vi "reward_behavior_michelle_visjitter_conswinadaptive_enticefx.vi"() -> ()   [LabVIEW 2019]
doc: "The myRIO Project template acquires acceleration data from the onboard accelerometer and displays the changes of acceleration values in a waveform chart."
uses:
  <vilib>/Analysis/Matrix/Datatypes/RealMatrix.ctl
  <vilib>/myRIO/Common/Instrument Driver Framework/myRIO v1.0/Encoder/typedefs/Encoder Signal Mode.ctl
  <vilib>/myRIO/Instrument Drivers/Onboard IO/Encoder/typedefs/Encoder Reference.ctl
  <vilib>/myRIO/Common/Instrument Driver Framework/Utilities/typedefs/myRIO Generic Hardware Reference.ctl
  <vilib>/myRIO/Common/Instrument Driver Framework/Utilities/typedefs/Hardware Version Enum.ctl
  <vilib>/myRIO/Common/Instrument Driver Framework/Utilities/typedefs/myRIO v1.0 Reference.ctl
  <vilib>/myRIO/Common/Instrument Driver Framework/Utilities/typedefs/Generic FPGA Reference.ctl
  <vilib>/myRIO/Common/Instrument Driver Framework/myRIO v1.0/Encoder/typedefs/Encoder Channels Enum.ctl
  <vilib>/myRIO/Common/Instrument Driver Framework/myRIO v1.0/Encoder/typedefs/Encoder Configuration v1.0.ctl
  <vilib>/userdefined/High Color/nirio_resource_hc.ctl
  <vilib>/myRIO/Instrument Drivers/Onboard IO/DIO/typedefs/DIO Reference.ctl
  <vilib>/myRIO/Common/Instrument Driver Framework/myRIO v1.0/DIO/typedefs/DIO Channels List.ctl
  <vilib>/myRIO/Common/Instrument Driver Framework/myRIO v1.0/DIO/typedefs/DIO Channels Enum.ctl
  <vilib>/myRIO/Common/Instrument Driver Framework/Utilities/vis/Is FPGA Ref Available.vi
  <vilib>/myRIO/Common/Instrument Driver Framework/myRIO v1.0/Encoder/vis/myRIO v1.1 Open Encoder.vi
  <vilib>/myRIO/Instrument Drivers/Onboard IO/Encoder/vis/Read.vi
  <vilib>/myRIO/Common/Instrument Driver Framework/myRIO v1.0/DIO/vis/myRIO v1.1 Open DIO.vi
  <vilib>/myRIO/Instrument Drivers/Onboard IO/DIO/vis/Write.vi
  <vilib>/myRIO/Instrument Drivers/Onboard IO/DIO/vis/Read.vi
  <vilib>/myRIO/Common/Instrument Driver Framework/Utilities/vis/Validate Channels.vi
  <vilib>/myRIO/Common/Instrument Driver Framework/myRIO v1.0/Encoder/vis/myRIO v1.0 Reserve Encoder.vi
  <vilib>/myRIO/Common/Instrument Driver Framework/myRIO v1.0/DIO/vis/myRIO v1.0 Reserve DIO.vi
  <vilib>/myRIO/Common/Instrument Driver Framework/myRIO v1.0/Encoder/vis/myRIO v1.0 Build MUX Configuration Encoder.vi
  <vilib>/myRIO/Common/Instrument Driver Framework/myRIO v1.0/Resource Manager/vis/myRIO v1.0 Reserve Channel List.vi
  <vilib>/myRIO/Common/Instrument Driver Framework/myRIO v1.0/DIO/vis/myRIO v1.0 Build MUX Configuration DIO.vi
  <vilib>/myRIO/Common/Instrument Driver Framework/myRIO v1.0/Resource Manager/vis/myRIO v1.0 Create Configuration List.vi
  <vilib>/myRIO/Common/Instrument Driver Framework/myRIO v1.0/Resource Manager/vis/myRIO v1.0 Reserve Channel.vi
  <vilib>/myRIO/Common/Instrument Driver Framework/myRIO v1.0/Resource Manager/vis/myRIO v1.0 Unreserve Channel.vi
  <vilib>/myRIO/Common/Instrument Driver Framework/myRIO v1.0/Resource Manager/vis/myRIO v1.0 Build Mutex Name.vi
  <vilib>/Utility/VariantDataType/GetNumericInfo.vi
  <vilib>/Utility/error.llb/Error Cluster From Error Code.vi
  <vilib>/myRIO/Common/Instrument Driver Framework/myRIO v1.0/myRIO v1.1 Open.vi
  <vilib>/myRIO/Common/Instrument Driver Framework/Utilities/vis/IO Manager.vi
  <vilib>/myRIO/Common/Instrument Driver Framework/Utilities/vis/Configuration Manager.vi
  <vilib>/myRIO/Common/Instrument Driver Framework/myRIO v1.0/Resource Manager/vis/myRIO v1.0 Configure IO.vi
  <vilib>/myRIO/Common/Instrument Driver Framework/myRIO v1.0/myRIO v1.0 Close.vi
  <vilib>/myRIO/Common/Instrument Driver Framework/myRIO v1.0/Encoder/vis/myRIO v1.0 Configure Encoder.vi
  <vilib>/myRIO/Common/Instrument Driver Framework/myRIO v1.0/Encoder/vis/myRIO v1.0 Read Encoder.vi
  <vilib>/myRIO/Common/Instrument Driver Framework/myRIO v1.0/DIO/vis/myRIO v1.0 Read DIO.vi
  <vilib>/myRIO/Common/Instrument Driver Framework/myRIO v1.0/DIO/vis/myRIO v1.0 Write DIO.vi
  <vilib>/myRIO/Express VI/Onboard IO/Encoder/Encoder Express VI.xnode
  <vilib>/myRIO/Instrument Drivers/Onboard IO/Encoder/vis/myRIO Encoder Open.xnode
  <vilib>/myRIO/Express VI/Onboard IO/DI/DI Express VI.xnode
  <vilib>/myRIO/Instrument Drivers/Onboard IO/DIO/vis/myRIO DIO Open.xnode
  <vilib>/myRIO/Express VI/Onboard IO/DO/DO Express VI.xnode
  <vilib>/myRIO/Instrument Drivers/Onboard IO/Encoder/Encoder.lvlib
  <vilib>/myRIO/Instrument Drivers/Onboard IO/DIO/DIO.lvlib
  <vilib>/Analysis/Matrix/NI_Matrix.lvlib
panel:
  out "Enticements":i32
  in  "Entice":bool
  out "Misses":i32
  out "GoAhead":bool
  out "TimeOutDuration":i32
  out "ActiveTime":dbl
  out "ConsumptionGo":bool=TRUE
  out "Consumption_Period":i32
  out "Watch_Display":bool=TRUE
  in  "Give reward":bool
  out "Timings":dbl[](array[numeric])
  out "ISI":dbl
  out "ISI start time":dbl
  out "Time_out":bool=TRUE
  out "Time since lick":dbl
  out "Time of last lick":dbl
  out "Rewarded trials":dbl[](array[numeric])
  out "Rewards":u16
  out "Active Trial":bool
  out "Array temp2":T1
  out "Stimuli Loaded":bool
  out "Stim_ID":dbl[](array[numeric])
  out "Reward_mat":dbl[](array[numeric])
  out "Reward":bool=TRUE
  out "Frame clock":i32
  out "Licks":u32
  out "Lick":bool
  out "Time":dbl
  out "Stop":bool
  in  "Frames to collect":u32
  out "Overflow?":bool
  out "Counter Value":i32
  out "Velocity":dbl
  out "Velocity Plot":dbl[](graph)
  out "Velocity array":dbl[](array[numeric])
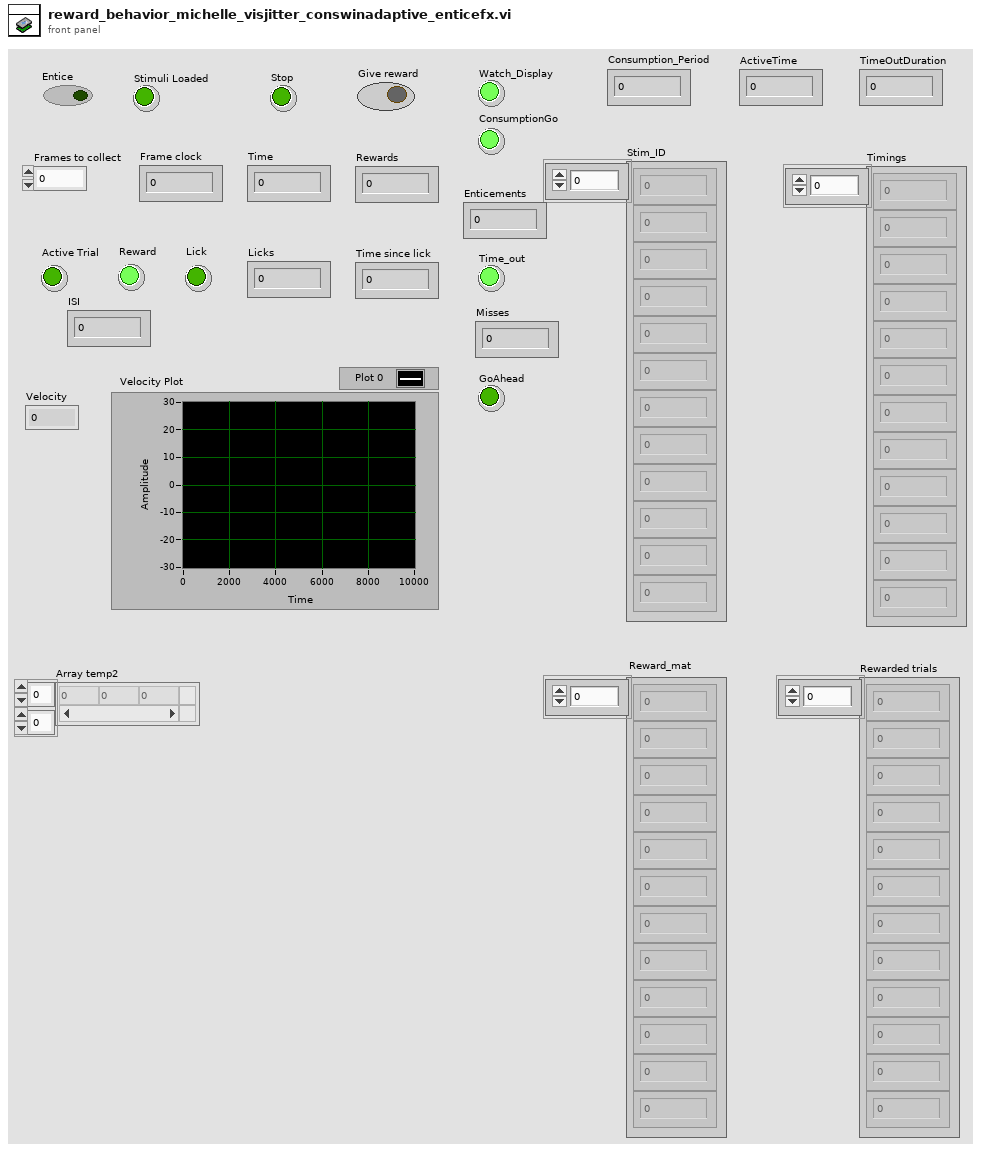
[diagram p1: front panel]
types:
  T1 = typedef "NI_Matrix.lvlib/RealMatrix.ctl" = dbl[][]
  T2 = typedef "Encoder.lvlib/Encoder Reference.ctl" = cluster{"myRIO Reference":T3, "Encoder Channels Enum":T7}
  T3 = typedef "myRIO Generic Hardware Reference.ctl" = cluster{"myRIO Model":T4, "myRIO Hardware Reference":T5}
  T4 = typedef "Hardware Version Enum.ctl" = enum16{"Unknown", "myRIO-1900", "myRIO-1950", "roboRIO", "NI ELVIS RIO CM", "ELVIS III"}
  T5 = typedef "myRIO v1.0 Reference.ctl" = cluster{"Generic FPGA Reference":T6, "Allow multiple opens":bool}
  T6 = typedef "Generic FPGA Reference.ctl" = refnum<k20>
  T7 = typedef "Encoder Channels Enum.ctl" = enum16{"Not Connected", "C/ENC0", "C/ENC1", "A/ENC", "A/ENC0", "A/ENC1", "A/ENC2", "A/ENC3", "A/ENC4", "A/ENC5", "A/ENC6", "A/ENC7", "A/ENC8", "A/ENC9", "B/ENC", "B/ENC0", "B/ENC1", "B/ENC2", "B/ENC3", "B/ENC4", "B/ENC5", "B/ENC6", "B/ENC7", "B/ENC8", "B/ENC9", "DIO/ENC0", "DIO/ENC1", "DIO/ENC2", "DIO/ENC3", "DIO/ENC4"}
  T8 = typedef "Encoder Signal Mode.ctl" = enum16{"Quadrature phase signal", "Step and direction signal"}
  T9 = typedef "nirio_resource_hc.ctl" = tag
  T10 = typedef "DIO.lvlib/DIO Reference.ctl" = cluster{"myRIO Reference":T3, "DIO Channels List":T11}
  T11 = typedef "DIO Channels List.ctl" = T12[]
  T12 = typedef "DIO Channels Enum.ctl" = enum16{"Not Connected", "C/DIO0", "C/DIO1", "C/DIO2", "C/DIO3", "C/DIO4", "C/DIO5", "C/DIO6", "C/DIO7", "A/DIO0", "A/DIO1", "A/DIO2", "A/DIO3", "A/DIO4", "A/DIO5", "A/DIO6", "A/DIO7", "A/DIO8", "A/DIO9", "A/DIO10", "A/DIO11", "A/DIO12", "A/DIO13", "A/DIO14", "A/DIO15", "A/DIO16", "A/DIO17", "A/DIO18", "A/DIO19", "B/DIO0", "B/DIO1", "B/DIO2", "B/DIO3", "B/DIO4", "B/DIO5", "B/DIO6", "B/DIO7", "B/DIO8", "B/DIO9", "B/DIO10", "B/DIO11", "B/DIO12", "B/DIO13", "B/DIO14", "B/DIO15", "B/DIO16", "B/DIO17", "B/DIO18", "B/DIO19", "LED0", "LED1", "LED2", "LED3", "Button0", "DIO/DIO0", "DIO/DIO1", "DIO/DIO2", "DIO/DIO3", "DIO/DIO4", "DIO/DIO5", "DIO/DIO6", "DIO/DIO7", "DIO/DIO8", "DIO/DIO9", "SPI/CS0", "SPI/CS1", "SPI/CS2", "SPI/CS3", "LED RADIO (Green)", "LED RADIO (Red)", "LED COMM (Green)", "LED COMM (Red)", "LED MODE (Green)", "LED MODE (Red)"}
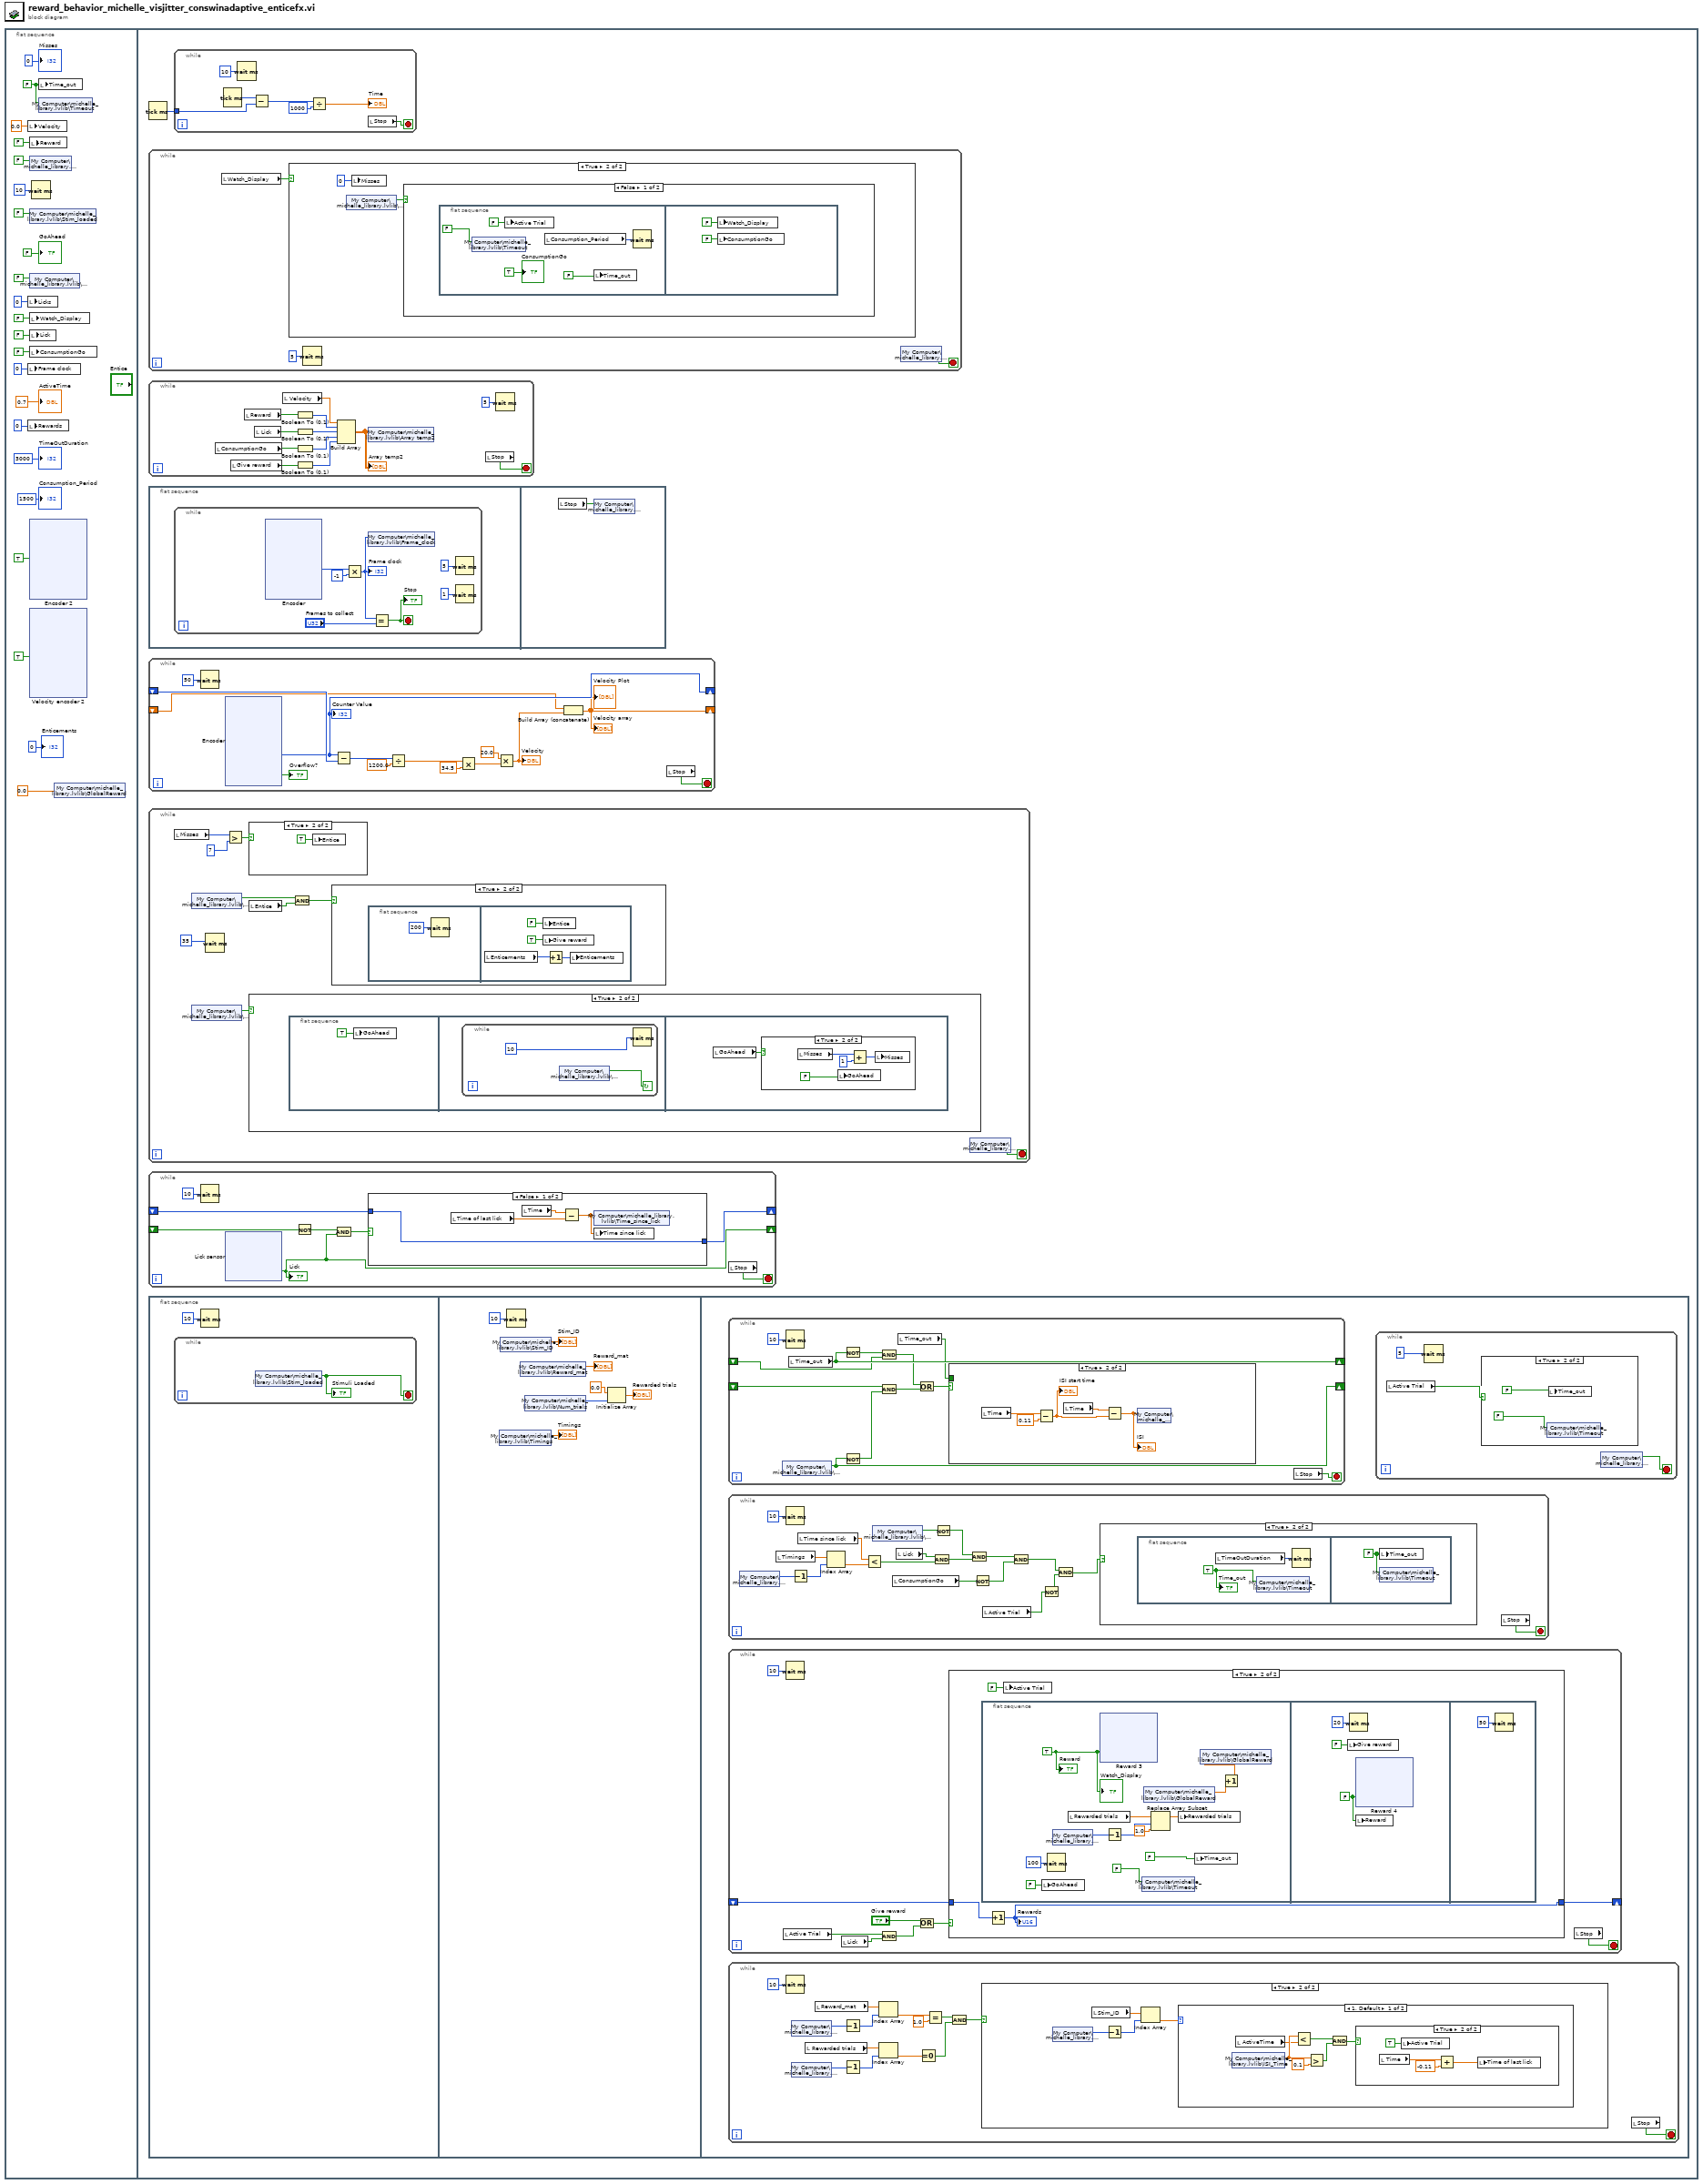
[diagram p0: block diagram]
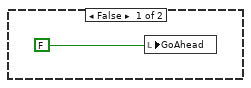
[diagram p4: hidden frame]
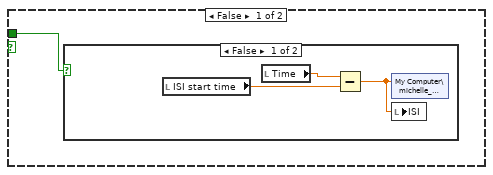
[diagram p10: hidden frame]
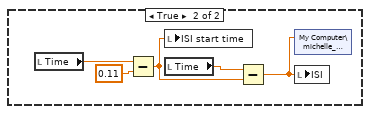
[diagram p11: hidden frame]
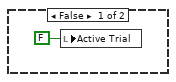
[diagram p12: hidden frame]
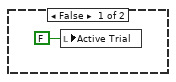
[diagram p13: hidden frame]
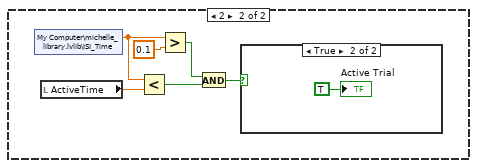
[diagram p14: hidden frame]
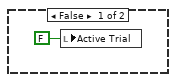
[diagram p15: hidden frame]
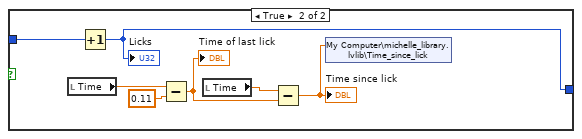
[diagram p17: hidden frame]
diagram:
  n1 = flat-sequence {
    frame #0 {
      w10 = FALSE ("Time_out")
      n2 = local write "Velocity"(0.0 ("Velocity")) -> ()
      n3 = local write "Licks"(u32 0 ("Licks")) -> ()
      n4 = local write "Frame clock"(u32 0 ("Frames")) -> ()
      n5 = local write "Rewards"(u16 0 ("Rewards")) -> ()
      n6 = local write "Reward"(FALSE ("Give reward")) -> ()
      n7 = shared-variable "My Computer\\michelle_library.lvlib\\Stop"(FALSE ("Stop")) -> ()  [unwired: 1 in, 1 out]
      n8 = shared-variable "My Computer\\michelle_library.lvlib\\Stim_loaded"(FALSE ("Stim_loaded")) -> ()  [unwired: 1 in, 1 out]
      n9 = shared-variable "My Computer\\michelle_library.lvlib\\Display"(FALSE ("Display")) -> ()  [unwired: 1 in, 1 out]
      n10 = local write "Watch_Display"(FALSE ("Watch_Display")) -> ()
      n11 = local write "Lick"(FALSE ("Lick")) -> ()
      n12 = local write "ConsumptionGo"(FALSE ("ConsumptionGo")) -> ()
      n13 = xnode "Encoder 2"("Reset Counter"=TRUE) -> ()  [unwired: 1 in, 4 out]
      n14 = xnode "Velocity encoder 2"("Reset Counter"=TRUE) -> ()  [unwired: 1 in, 4 out]
      n15 = Wait (ms)(milliseconds to wait=u32 10) -> ()  [unwired: 1 out]
      n16 = local write "Time_out"(w10) -> ()
      n17 = shared-variable "My Computer\\michelle_library.lvlib\\Timeout"(w10) -> ()  [unwired: 1 in, 1 out]
      n18 = shared-variable "My Computer\\michelle_library.lvlib\\GlobalReward"(0.0) -> ()  [unwired: 1 in, 1 out]
      "Consumption_Period" <- 1500
      "ActiveTime" <- 0.7
      "TimeOutDuration" <- 3000
      "GoAhead" <- FALSE
      "Misses" <- 0
      "Enticements" <- 0
    }
    frame #1 {
      n19 = Tick Count (ms)() -> (millisecond timer value=w115:u32)
      n20 = while {
        stop <- w142 stop-if-true
        n21 = local read "Watch_Display"() -> (w141:bool)
        n22 = case shown="True" w141 {
          frame False {
          }
          frame True {
            n23 = shared-variable "My Computer\\michelle_library.lvlib\\Display"() -> (w144:bool)  [unwired: 1 in, 1 out]
            n24 = local write "Misses"(0) -> ()
            n25 = case shown="False" w144 {
              frame False {
                n26 = flat-sequence {
                  frame #0 {
                    n27 = shared-variable "My Computer\\michelle_library.lvlib\\Timeout"(FALSE) -> ()  [unwired: 1 in, 1 out]
                    n28 = local write "Active Trial"(FALSE) -> ()
                    n29 = local read "Consumption_Period"() -> (w149:i32)
                    n30 = local write "Time_out"(FALSE) -> ()
                    n31 = Wait (ms)(milliseconds to wait=w149) -> ()  [unwired: 1 out]
                    "ConsumptionGo" <- TRUE
                  }
                  frame #1 {
                    n32 = local write "Watch_Display"(FALSE ("Watch_Display")) -> ()
                    n33 = local write "ConsumptionGo"(FALSE ("ConsumptionGo")) -> ()
                  }
                }
              }
              frame True {
              }
            }
          }
        }
        n34 = Wait (ms)(milliseconds to wait=u32 5) -> ()  [unwired: 1 out]
        n35 = shared-variable "My Computer\\michelle_library.lvlib\\Stop"() -> (w142:bool)  [unwired: 1 in, 1 out]
      }
      n36 = while {
        stop <- w157 stop-if-true
        n37 = local read "ConsumptionGo"() -> (w155:bool)
        n38 = local read "Give reward"() -> (w154:bool)
        n39 = local read "Reward"() -> (w162:bool)
        n40 = local read "Lick"() -> (w163:bool)
        n41 = local read "Velocity"() -> (w161:dbl)
        n42 = Boolean To (0,1)(Boolean=w162) -> (0, 1=w160:i16)
        n43 = Boolean To (0,1)(Boolean=w163) -> (0, 1=w159:i16)
        n44 = Boolean To (0,1)(Boolean=w155) -> (0, 1=w153:i16)
        n45 = Boolean To (0,1)(Boolean=w154) -> (0, 1=w152:i16)
        n46 = Build Array(w161, w160, w159, w153, w152) -> (w156:T1)
        "Array temp2" <- w156
        n47 = shared-variable "My Computer\\michelle_library.lvlib\\Array temp2"(w156) -> ()  [unwired: 1 in, 1 out]
        n48 = local read "Stop"() -> (w157:bool)
        n49 = Wait (ms)(milliseconds to wait=u32 5) -> ()  [unwired: 1 out]
      }
      n50 = flat-sequence {
        frame #0 {
          n51 = while {
            stop <- w364 stop-if-true
            n52 = xnode "Encoder"() -> ("Counter Value"=w368:i32)  [unwired: 2 in, 3 out]
            n53 = Multiply(x=w368, y=-1) -> (x*y=w363:i32)
            "Frame clock" <- w363
            n54 = shared-variable "My Computer\\michelle_library.lvlib\\Frame_clock"(w363) -> ()  [unwired: 1 in, 1 out]
            n55 = Equal?(x=w363, y="Frames to collect") -> (x = y?=w364:bool)
            "Stop" <- w364
            n56 = Wait (ms)(milliseconds to wait=u32 5) -> ()  [unwired: 1 out]
            n57 = Wait (ms)(milliseconds to wait=u32 1) -> ()  [unwired: 1 out]
          }
        }
        frame #1 {
          n58 = local read "Stop"() -> (w416:bool)
          n59 = shared-variable "My Computer\\michelle_library.lvlib\\Stop"(w416) -> ()  [unwired: 1 in, 1 out]
        }
      }
      n60 = while {
        shift-right: [w481] -> _
        shift-left: _ -> [w482]
        shift-right: [w473] -> _
        shift-left: _ -> [w472]
        stop <- w471 stop-if-true
        n61 = Wait (ms)(milliseconds to wait=u32 50) -> ()  [unwired: 1 out]
        n62 = xnode "Encoder"() -> ("Counter Value"=w481:i32, "Overflow?"=→"Overflow?":bool)  [unwired: 2 in, 2 out]
        "Counter Value" <- w481
        n63 = Subtract(x=w481, y=w482) -> (x-y=w474:i32)
        n64 = Divide(x=w474, y=1200.0 ("600")) -> (x/y=w479:dbl)
        n65 = Multiply(x=w479, y=34.5) -> (x*y=w477:dbl)
        n66 = Multiply(x=20.0, y=w477) -> (x*y=w475:dbl)
        "Velocity" <- w475
        n67 = Build Array (concatenate)(w472, w475) -> (w473:dbl[])
        "Velocity Plot" <- w473
        "Velocity array" <- w473
        n68 = local read "Stop"() -> (w471:bool)
      }
      n69 = while {
        stop <- w124 stop-if-true
        n70 = local read "Misses"() -> (w122:i32)
        n71 = shared-variable "My Computer\\michelle_library.lvlib\\Display"() -> (w118:bool)  [unwired: 1 in, 1 out]
        n72 = shared-variable "My Computer\\michelle_library.lvlib\\Display"() -> (w123:bool)  [unwired: 1 in, 1 out]
        n73 = Wait (ms)(milliseconds to wait=35) -> ()  [unwired: 1 out]
        n74 = Greater?(x=w122, y=7) -> (0:w120:bool)
        n75 = case shown="True" w120 {
          frame False {
          }
          frame True {
            n76 = local write "Entice"(TRUE) -> ()
          }
        }
        n77 = local read "Entice"() -> (w117:bool)
        n78 = case shown="True" w123 {
          frame False {
            n79 = local write "GoAhead"(FALSE) -> ()
          }
          frame True {
            n80 = flat-sequence {
              frame #0 {
                n81 = local write "GoAhead"(TRUE) -> ()
              }
              frame #1 {
                n82 = while {
                  stop <- w134 continue-if-true
                  n83 = shared-variable "My Computer\\michelle_library.lvlib\\Display"() -> (w134:bool)  [unwired: 1 in, 1 out]
                  n84 = Wait (ms)(milliseconds to wait=10) -> ()  [unwired: 1 out]
                }
              }
              frame #2 {
                n85 = local read "GoAhead"() -> (w135:bool)
                n86 = case shown="True" w135 {
                  frame False {
                  }
                  frame True {
                    n87 = local read "Misses"() -> (w139:i32)
                    n88 = local write "GoAhead"(FALSE) -> ()
                    n89 = Add(x=w139, y=1) -> (x+y=w137:i32)
                    n90 = local write "Misses"(w137) -> ()
                  }
                }
              }
            }
          }
        }
        n91 = And(x=w118, y=w117) -> (x .and. y?=w119:bool)
        n92 = case shown="True" w119 {
          frame False {
          }
          frame True {
            n93 = flat-sequence {
              frame #0 {
                n94 = Wait (ms)(milliseconds to wait=200) -> ()  [unwired: 1 out]
              }
              frame #1 {
                n95 = local read "Enticements"() -> (w127:i32)
                n96 = local write "Entice"(FALSE) -> ()
                n97 = local write "Give reward"(TRUE) -> ()
                n98 = Increment(x=w127) -> (x+1=w126:i32)
                n99 = local write "Enticements"(w126) -> ()
              }
            }
          }
        }
        n100 = shared-variable "My Computer\\michelle_library.lvlib\\Stop"() -> (w124:bool)  [unwired: 1 in, 1 out]
      }
      n101 = while {
        shift-right: [w423] -> _
        shift-left: _ -> [w422]
        shift-right: [w417] -> _
        shift-left: _ -> [w420]
        stop <- w421 stop-if-true
        n102 = Wait (ms)(milliseconds to wait=u32 10) -> ()  [unwired: 1 out]
        n103 = xnode "Lick sensor"() -> ("C/DIO1 (DIO1)"=w417:bool)  [unwired: 1 in, 1 out]
        "Lick" <- w417
        n104 = Not(x=w420) -> (.not. x?=w419:bool)
        n105 = And(x=w419, y=w417) -> (x .and. y?=w418:bool)
        n106 = case shown="False" w418 {
          tunnel: [w428 w435] -> w423
          tunnel: w422 -> [w428 w434]
          frame False {
            n107 = local read "Time of last lick"() -> (w426:dbl)
            n108 = local read "Time"() -> (w427:dbl)
            n109 = Subtract(x=w427, y=w426) -> (x-y=w425:dbl)
            n110 = shared-variable "My Computer\\michelle_library.lvlib\\Time_since_lick"(w425) -> ()  [unwired: 1 in, 1 out]
            n111 = local write "Time since lick"(w425) -> ()
          }
          frame True {
            n112 = local read "Time"() -> (w431:dbl)
            n113 = Increment(x=w434) -> (x+1=w435:u32)
            "Licks" <- w435
            n114 = Subtract(x=w431, y=0.11) -> (x-y=w429:dbl)
            "Time of last lick" <- w429
            n115 = local read "Time"() -> (w433:dbl)
            n116 = Subtract(x=w433, y=w429) -> (x-y=w432:dbl)
            "Time since lick" <- w432
            n117 = shared-variable "My Computer\\michelle_library.lvlib\\Time_since_lick"(w432) -> ()  [unwired: 1 in, 1 out]
          }
        }
        n118 = local read "Stop"() -> (w421:bool)
      }
      n119 = flat-sequence {
        frame #0 {
          n120 = while {
            stop <- w165 stop-if-true
            n121 = shared-variable "My Computer\\michelle_library.lvlib\\Stim_loaded"() -> (w165:bool)  [unwired: 1 in, 1 out]
            "Stimuli Loaded" <- w165
          }
          n122 = Wait (ms)(milliseconds to wait=u32 10) -> ()  [unwired: 1 out]
        }
        frame #1 {
          n123 = shared-variable "My Computer\\michelle_library.lvlib\\Timings"() -> (→"Timings":dbl[])  [unwired: 1 in, 1 out]
          n124 = shared-variable "My Computer\\michelle_library.lvlib\\Stim_ID"() -> (→"Stim_ID":dbl[])  [unwired: 1 in, 1 out]
          n125 = Wait (ms)(milliseconds to wait=u32 10) -> ()  [unwired: 1 out]
          n126 = shared-variable "My Computer\\michelle_library.lvlib\\Reward_mat"() -> (→"Reward_mat":dbl[])  [unwired: 1 in, 1 out]
          n127 = shared-variable "My Computer\\michelle_library.lvlib\\Num_trials"() -> (w169:u32)  [unwired: 1 in, 1 out]
          n128 = Initialize Array(0.0 ("element"), w169) -> (→"Rewarded trials":dbl[])
        }
        frame #2 {
          n129 = while {
            shift-right: [w210] -> _
            shift-left: _ -> [w208]
            shift-right: [w206] -> _
            shift-left: _ -> [w205]
            stop <- w211 stop-if-true
            n130 = shared-variable "My Computer\\michelle_library.lvlib\\Display"() -> (w206:bool)  [unwired: 1 in, 1 out]
            n131 = Wait (ms)(milliseconds to wait=u32 10) -> ()  [unwired: 1 out]
            n132 = local read "Time_out"() -> (w210:bool)
            n133 = Not(x=w210) -> (.not. x?=w209:bool)
            n134 = Not(x=w206) -> (.not. x?=w204:bool)
            n135 = And(x=w209, y=w208) -> (x .and. y?=w203:bool)
            n136 = And(x=w205, y=w204) -> (x .and. y?=w202:bool)
            n137 = local read "Time_out"() -> (w207:bool)
            n138 = Or(x=w203, y=w202) -> (x .or. y?=w201:bool)
            n139 = case shown="True" w201 {
              tunnel: w207 -> [w212 _]
              frame False {
                n140 = case shown="False" w212 {
                  frame False {
                    n141 = local read "ISI start time"() -> (w215:dbl)
                    n142 = local read "Time"() -> (w214:dbl)
                    n143 = Subtract(x=w214, y=w215) -> (x-y=w213:dbl)
                    n144 = shared-variable "My Computer\\michelle_library.lvlib\\ISI"(w213) -> ()  [unwired: 1 in, 1 out]
                    n145 = local write "ISI"(w213) -> ()
                  }
                  frame True {
                    n146 = local read "Time"() -> (w220:dbl)
                    n147 = Subtract(x=w220, y=0.11) -> (x-y=w217:dbl)
                    n148 = local write "ISI start time"(w217) -> ()
                    n149 = local read "Time"() -> (w218:dbl)
                    n150 = Subtract(x=w218, y=w217) -> (x-y=w216:dbl)
                    n151 = shared-variable "My Computer\\michelle_library.lvlib\\ISI"(w216) -> ()  [unwired: 1 in, 1 out]
                    n152 = local write "ISI"(w216) -> ()
                  }
                }
              }
              frame True {
                n153 = local read "Time"() -> (w225:dbl)
                n154 = Subtract(x=w225, y=0.11) -> (x-y=w222:dbl)
                "ISI start time" <- w222
                n155 = local read "Time"() -> (w223:dbl)
                n156 = Subtract(x=w223, y=w222) -> (x-y=w221:dbl)
                "ISI" <- w221
                n157 = shared-variable "My Computer\\michelle_library.lvlib\\ISI"(w221) -> ()  [unwired: 1 in, 1 out]
              }
            }
            n158 = local read "Stop"() -> (w211:bool)
          }
          n159 = while {
            stop <- w196 stop-if-true
            n160 = shared-variable "My Computer\\michelle_library.lvlib\\Trial"() -> (w186:u32)  [unwired: 1 in, 1 out]
            n161 = local read "Timings"() -> (w188:dbl[])
            n162 = Wait (ms)(milliseconds to wait=u32 10) -> ()  [unwired: 1 out]
            n163 = Decrement(x=w186) -> (x-1=w185:u32)
            n164 = local read "Time since lick"() -> (w195:dbl)
            n165 = Index Array(array=w188, index=w185) -> (element=w187:dbl)
            n166 = Less?(x=w195, y=w187) -> (x < y?=w194:bool)
            n167 = shared-variable "My Computer\\michelle_library.lvlib\\Display"() -> (w191:bool)  [unwired: 1 in, 1 out]
            n168 = local read "ConsumptionGo"() -> (w183:bool)
            n169 = local read "Lick"() -> (w193:bool)
            n170 = And(x=w193, y=w194) -> (x .and. y?=w189:bool)
            n171 = Not(x=w191) -> (.not. x?=w190:bool)
            n172 = And(x=w190, y=w189) -> (x .and. y?=w182:bool)
            n173 = Not(x=w183) -> (.not. x?=w184:bool)
            n174 = local read "Active Trial"() -> (w178:bool)
            n175 = And(x=w182, y=w184) -> (x .and. y?=w180:bool)
            n176 = Not(x=w178) -> (.not. x?=w181:bool)
            n177 = And(x=w180, y=w181) -> (x .and. y?=w179:bool)
            n178 = case shown="True" w179 {
              frame False {
              }
              frame True {
                n179 = flat-sequence {
                  frame #0 {
                    w198 = TRUE
                    n180 = local read "TimeOutDuration"() -> (w197:i32)
                    n181 = shared-variable "My Computer\\michelle_library.lvlib\\Timeout"(w198) -> ()  [unwired: 1 in, 1 out]
                    n182 = Wait (ms)(milliseconds to wait=w197) -> ()  [unwired: 1 out]
                    "Time_out" <- w198
                  }
                  frame #1 {
                    w199 = FALSE ("Timeout")
                    n183 = local write "Time_out"(w199) -> ()
                    n184 = shared-variable "My Computer\\michelle_library.lvlib\\Timeout"(w199) -> ()  [unwired: 1 in, 1 out]
                  }
                }
              }
            }
            n185 = local read "Stop"() -> (w196:bool)
          }
          n186 = while {
            shift-right: [w270] -> _
            shift-left: _ -> [w269]
            stop <- w272 stop-if-true
            n187 = local read "Active Trial"() -> (w267:bool)
            n188 = Wait (ms)(milliseconds to wait=u32 10) -> ()  [unwired: 1 out]
            n189 = local read "Lick"() -> (w268:bool)
            n190 = And(x=w267, y=w268) -> (x .and. y?=w266:bool)
            n191 = Or(x="Give reward", y=w266) -> (x .or. y?=w265:bool)
            n192 = case shown="True" w265 {
              tunnel: [w273 w276] -> w270
              tunnel: w269 -> [w273 w275]
              frame False {
              }
              frame True {
                n193 = flat-sequence {
                  frame #0 {
                    w287 = TRUE ("C/DIO0 (DIO0)")
                    n194 = local write "GoAhead"(FALSE) -> ()
                    n195 = Wait (ms)(milliseconds to wait=u32 100) -> ()  [unwired: 1 out]
                    n196 = shared-variable "My Computer\\michelle_library.lvlib\\Trial"() -> (w286:u32)  [unwired: 1 in, 1 out]
                    n197 = local read "Rewarded trials"() -> (w284:dbl[])
                    n198 = xnode "Reward 3"("C/DIO0 (DIO0)"=w287) -> ()  [unwired: 1 in, 1 out]
                    n199 = Decrement(x=w286) -> (x-1=w285:u32)
                    n200 = shared-variable "My Computer\\michelle_library.lvlib\\Timeout"(FALSE) -> ()  [unwired: 1 in, 1 out]
                    n201 = shared-variable "My Computer\\michelle_library.lvlib\\GlobalReward"() -> (w278:dbl)  [unwired: 1 in, 1 out]
                    n202 = Replace Array Subset(array=w284, new element=1.0 ("new element/subarray"), index=w285) -> (w282:dbl[])
                    n203 = local write "Rewarded trials"(w282) -> ()
                    n204 = local write "Time_out"(FALSE) -> ()
                    n205 = Increment(x=w278) -> (x+1=w277:dbl)
                    n206 = shared-variable "My Computer\\michelle_library.lvlib\\GlobalReward"(w277) -> ()  [unwired: 1 in, 1 out]
                    "Reward" <- w287
                    "Watch_Display" <- w287
                  }
                  frame #1 {
                    w326 = FALSE ("C/DIO0 (DIO0)")
                    n207 = local write "Give reward"(FALSE ("Give reward")) -> ()
                    n208 = Wait (ms)(milliseconds to wait=u32 20) -> ()  [unwired: 1 out]
                    n209 = xnode "Reward 4"("C/DIO0 (DIO0)"=w326) -> ()  [unwired: 1 in, 1 out]
                    n210 = local write "Reward"(w326) -> ()
                  }
                  frame #2 {
                    n211 = Wait (ms)(milliseconds to wait=u32 50) -> ()  [unwired: 1 out]
                  }
                }
                n212 = Increment(x=w275) -> (x+1=w276:u16)
                "Rewards" <- w276
                n213 = local write "Active Trial"(FALSE ("Active Trial")) -> ()
              }
            }
            n214 = local read "Stop"() -> (w272:bool)
          }
          n215 = while {
            stop <- w239 stop-if-true
            n216 = Wait (ms)(milliseconds to wait=u32 10) -> ()  [unwired: 1 out]
            n217 = shared-variable "My Computer\\michelle_library.lvlib\\Trial"() -> (w235:u32)  [unwired: 1 in, 1 out]
            n218 = shared-variable "My Computer\\michelle_library.lvlib\\Trial"() -> (w231:u32)  [unwired: 1 in, 1 out]
            n219 = local read "Rewarded trials"() -> (w232:dbl[])
            n220 = local read "Reward_mat"() -> (w234:dbl[])
            n221 = Decrement(x=w235) -> (x-1=w236:u32)
            n222 = Decrement(x=w231) -> (x-1=w230:u32)
            n223 = Index Array(array=w234, index=w236) -> (element=w237:dbl)
            n224 = Index Array(array=w232, index=w230) -> (element=w229:dbl)
            n225 = Equal To 0?(x=w229) -> (x = 0?=w228:bool)
            n226 = Equal?(x=w237, y=1.0) -> (x = y?=w227:bool)
            n227 = And(x=w227, y=w228) -> (x .and. y?=w226:bool)
            n228 = case shown="True" w226 {
              frame False {
                n229 = local write "Active Trial"(FALSE ("Active_trial")) -> ()
              }
              frame True {
                n230 = shared-variable "My Computer\\michelle_library.lvlib\\Trial"() -> (w242:u32)  [unwired: 1 in, 1 out]
                n231 = local read "Stim_ID"() -> (w244:dbl[])
                n232 = Decrement(x=w242) -> (x-1=w243:u32)
                n233 = Index Array(array=w244, index=w243) -> (element=w241:dbl)
                n234 = case shown="1, Default" w241 {
                  frame 1, Default {
                    n235 = shared-variable "My Computer\\michelle_library.lvlib\\ISI_Time"() -> (w250:dbl)  [unwired: 1 in, 1 out]
                    n236 = local read "ActiveTime"() -> (w245:dbl)
                    n237 = Less?(x=w250, y=w245) -> (x < y?=w248:bool)
                    n238 = Greater?(x=w250, y=0.1) -> (0:w247:bool)
                    n239 = And(x=w248, y=w247) -> (x .and. y?=w246:bool)
                    n240 = case shown="True" w246 {
                      frame False {
                        n241 = local write "Active Trial"(FALSE ("Active Trial")) -> ()
                      }
                      frame True {
                        n242 = local read "Time"() -> (w254:dbl)
                        n243 = local write "Active Trial"(TRUE ("Active Trial")) -> ()
                        n244 = Add(x=w254, y=-0.11) -> (x+y=w252:dbl)
                        n245 = local write "Time of last lick"(w252) -> ()
                      }
                    }
                  }
                  frame 2 {
                    n246 = shared-variable "My Computer\\michelle_library.lvlib\\ISI_Time"() -> (w260:dbl)  [unwired: 1 in, 1 out]
                    n247 = local read "ActiveTime"() -> (w256:dbl)
                    n248 = Less?(x=w260, y=w256) -> (x < y?=w258:bool)
                    n249 = Greater?(x=w260, y=0.1) -> (0:w259:bool)
                    n250 = And(x=w259, y=w258) -> (x .and. y?=w257:bool)
                    n251 = case shown="True" w257 {
                      frame False {
                        n252 = local write "Active Trial"(FALSE ("Active Trial")) -> ()
                      }
                      frame True {
                        "Active Trial" <- TRUE ("Active Trial")
                      }
                    }
                  }
                }
              }
            }
            n253 = local read "Stop"() -> (w239:bool)
          }
          n254 = while {
            stop <- w175 stop-if-true
            n255 = local read "Active Trial"() -> (w174:bool)
            n256 = Wait (ms)(milliseconds to wait=5) -> ()  [unwired: 1 out]
            n257 = case shown="True" w174 {
              frame False {
              }
              frame True {
                n258 = shared-variable "My Computer\\michelle_library.lvlib\\Timeout"(FALSE) -> ()  [unwired: 1 in, 1 out]
                n259 = local write "Time_out"(FALSE) -> ()
              }
            }
            n260 = shared-variable "My Computer\\michelle_library.lvlib\\Stop"() -> (w175:bool)  [unwired: 1 in, 1 out]
          }
        }
      }
      n261 = while {
        tunnel: w115 -> [w536]
        stop <- w534 stop-if-true
        n262 = Tick Count (ms)() -> (millisecond timer value=w537:u32)
        n263 = Wait (ms)(milliseconds to wait=u32 10) -> ()  [unwired: 1 out]
        n264 = Subtract(x=w537, y=w536) -> (x-y=w533:u32)
        n265 = Divide(x=w533, y=u32 1000) -> (x/y=→"Time":dbl)
        n266 = local read "Stop"() -> (w534:bool)
      }
    }
  }
